vi "MVP Valve Wait.vi"(0 "VISA resource name":refnum<visa-resource-name>="VALVE", 7 "Valve # (1=a, 2=b, ....  0 = no prefix)":u8, 11 "error in (no error)":errorcluster) -> (4 "VISA resource name out":refnum<visa-resource-name>, 15 "error out":errorcluster)   [LabVIEW 2015]
doc: "Reads a response from the pump affter a command is sent\n\nModified from original which is Copyright 2005, National Instruments Corporation"
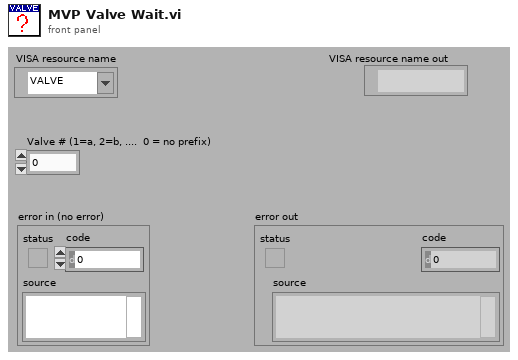
[diagram p1: front panel]
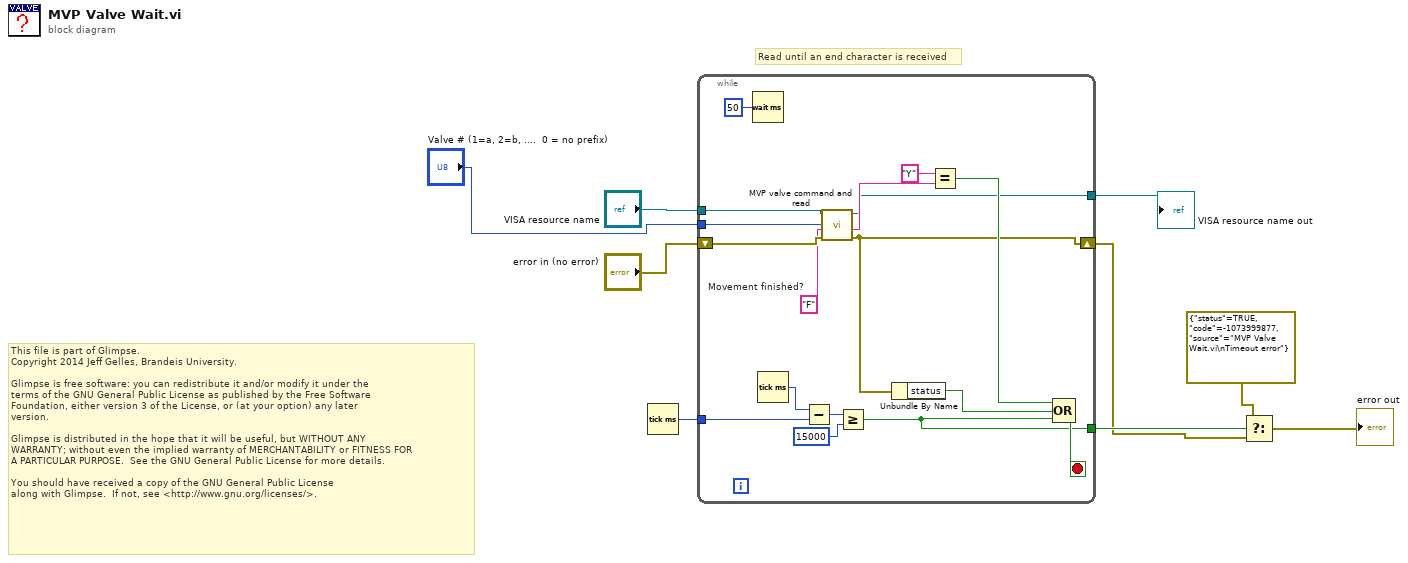
[diagram p0: block diagram]
diagram:
  # "This file is part of Glimpse. \nCopyright 2014 Jeff Gelles, Brandeis University.    \n\nGlimpse is free software: you can redistribute it and/or modify it under the \nterms of the GNU General Public License as published by the Free Software \nFoundation, either version 3 of the License, or (at your option) any later \nversion.\n\nGlimpse is distributed in the hope that it will be useful, but WITHOUT ANY \nWARRANTY; without even the implied warranty of MERCHANTABILITY or FITNESS FOR \nA PARTICULAR PURPOSE.  See the GNU General Public License for more details.\n\nYou should have received a copy of the GNU General Public License\nalong with Glimpse.  If not, see <http://www.gnu.org/licenses/>."
  # "Read until an end character is received"
  n1 = Tick Count (ms)() -> (millisecond timer value=w7:u32)
  n2 = while {
    tunnel: "VISA resource name" -> [w17]
    tunnel: [w10] -> w4
    tunnel: w7 -> [w24]
    tunnel: [w20] -> w6
    shift-right: [w11] -> w5
    shift-left: "error in (no error)" -> [w18]
    tunnel: "Valve # (1=a, 2=b, ....  0 = no prefix)" -> [w16]
    stop <- w21 stop-if-true
    w15 = "F"  # Movement finished?
    n3 = Wait (ms)(milliseconds to wait=u32 50) -> ()  [unwired: 1 out]
    n4 = Tick Count (ms)() -> (millisecond timer value=w25:u32)
    n5 = Subtract(x=w25, y=w24) -> (x-y=w23:u32)
    n6 = call "MVP valve command and read.vi"("error in"=w18, "command\n(w/o pump # prefix)"=w15, "Valve # (1=a, 2=b, ....  0 = no prefix)"=w16, "VISA resource name"=w17) -> ("error out"=w11:errorcluster, "Output String"=w14:string, "VISA resource name out"=w10:refnum<visa-resource-name>)  [unwired: 2 out]
    n7 = Greater Or Equal?(x=w23, y=u32 15000) -> (x >= y?=w20:bool)
    n8 = Unbundle By Name(w11) -> ("status"=w19:bool)
    n9 = Equal?(x="Y", y=w14) -> (x = y?=w12:bool)
    n10 = Compound Arithmetic op=OR(w12, w19, w20) -> (w21:bool)
  }
  "VISA resource name out" <- w4
  n11 = Select(t=errorcluster {"status"=TRUE, "code"=-1073999877, "source"="MVP Valve Wait.vi\nTimeout error"}, s=w6, f=w5) -> (s? t:f=→"error out":errorcluster)
